vi "CloseFile.vi"(8 "error in (no error)":errorcluster, 11 "file reference":refnum<file>) -> (0 "error out":errorcluster)   [LabVIEW 2017]
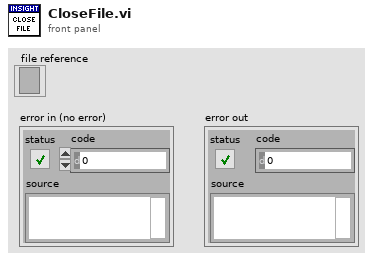
[diagram p1: front panel]
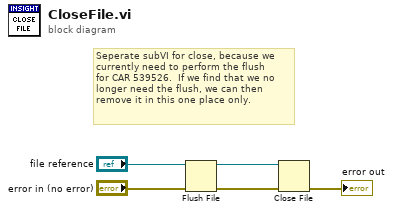
[diagram p0: block diagram]
diagram:
  # "Seperate subVI for close, because we\ncurrently need to perform the flush\nfor CAR 539526.  If we find that we no\nlonger need the flush, we can then \nremove it in this one place only."
  n1 = Flush File(refnum="file reference", error in="error in (no error)") -> (refnum out=w3:refnum<file>, error out=w5:errorcluster)
  n2 = Close File(refnum=w3, error in=w5) -> (error out=→"error out":errorcluster)  [unwired: 1 out]
